vi "SVT Fractional-octave Analysis (N Ch).vi"(0 "scaled signals [EU]":waveform(dbl)[](array[waveform])=[{"t0"=timestamp(0 s since 1904-01-01), "dt"=1.0, "Y"=[]}], 1 "restart averaging (F)":bool, 2 "reset filter (F)":bool, 5 "frequency range [Hz]":T8={"low frequency"=125.0, "high frequency"=8000.0} {"high frequency" min=0.001 format="%.2f"; "low frequency" min=0.001 format="%.2f"}, 7 "bandwidth":T2(ring)=enum."1/12 octave", 9 "dB On (T)":bool=TRUE, 11 "error in (no error)":errorcluster, 12 "averaging type":T9(ring), 13 "exp avg settings":T1={" mode"=enum."Fast", "time constant [ms]"=125.0} {"time constant [ms]" format="%.2f"}, 14 "equal confidence level [dB]":dbl=125.0 format="%.2f") -> (3 "filter settled":bool, 4 "octave spectra":T7(array[cluster]) {"band power" format="%.2f"; "nominal frequencies [Hz]" format="%.2f"}, 6 "unit labels":string[](array[string]), 8 "total band powers":dbl[](array[numeric]) format="%.2f", 10 "octave info":T3[](array[typedef]) {"engineering units" items=["custom..."=0, "V"=1, "A"=21, "C"=30, "pC"=31, "s"=32, "-"=29, "Pa"=2, "N"=20, "g"=3, "m/s^2"=4, "m/s"=5, "m"=6, "mm/s"=12, "mm"=13, "micron/s"=14, "micron"=15, "in/s^2"=7, "in/s"=8, "in"=9, "mil/s"=10, "mil"=11, "rad/s^2"=16, "rad/s"=17, "rad"=18, "deg/s^2"=26, "deg/s"=27, "deg"=28, "RPM"=22, "cycle/s^2"=23, "Hz"=24, "cycle"=25, "strain"=19]; "dB reference" format="%.2e"; "weighting filter" items=["Linear", "A-weighting", "B-weighting", "C-weighting", "ITU-R 468-4", "Dolby", "CCITT", "C-message", "Wb", "Wc", "Wd", "We", "Wf", "Wh", "Wj", "Wk", "Wm", "AES17 20 kHz lowpass", "AES17 40 kHz lowpass", "AES17 20 kHz highpass", "AES17 40 kHz highpass"]}, 15 "error out":errorcluster)   [LabVIEW 2017, in "SoundVib_Octave_2014 standard.lvlib"]
doc: "Performs a fractional-octave analysis on <B>scaled signal [EU]</B> in accordance with the IEC 61260:2014 and ANSI S1.11-2014 standards. Wire data to the <B>scaled signal [EU]</B> input to determine the polymorphic instance to use or manually select the instance."
uses:
  <vilib>/addons/Sound and Vibration/svt_Octave/SoundVib_Octave_2014 standard.lvlib
  <vilib>/addons/_NISVFA/_Shared subVIs/Controls/svc_Octave Info.ctl
  <vilib>/addons/_NISVFA/_Shared subVIs/Controls/svc_Octave Standard.ctl
  <vilib>/addons/_NISVFA/_Shared subVIs/Controls/svc_Weighting Filter Text Ring.ctl
  <vilib>/addons/_NISVFA/_Shared subVIs/Controls/svc_Engineering Units Text Ring.ctl
panel:
  out "# samples to settle":u64
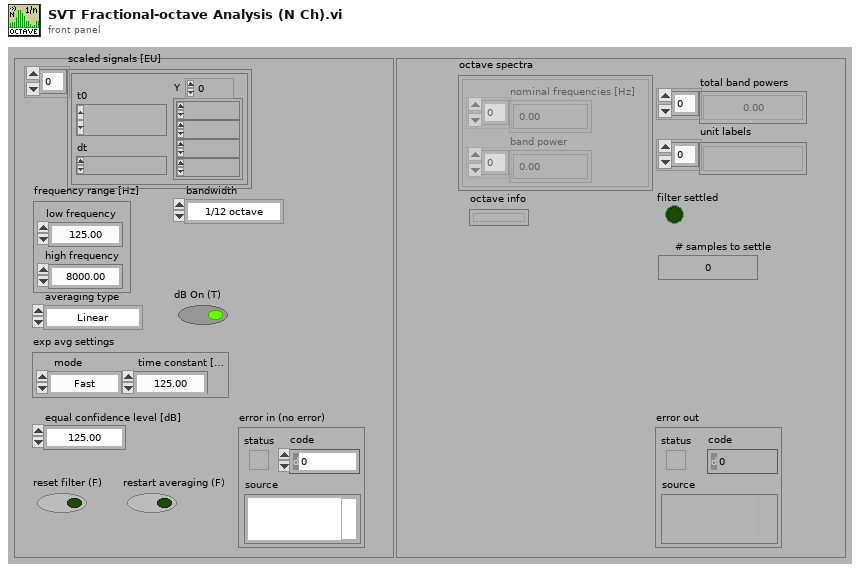
[diagram p1: front panel]
types:
  T1 = cluster{" mode":enum16{"Slow", "Fast", "Impulse", "Custom"}, "time constant [ms]":dbl}
  T2 = enum16{"1 octave", "1/3 octave", "1/6 octave", "1/12 octave", "1/24 octave"}
  T3 = typedef "svc_Octave Info.ctl" = cluster{"standard":T4, "bandwidth":enum16{"1 octave", "1/3 octave", "1/6 octave", "1/12 octave", "1/24 octave"}, "low band":i32, "high band":i32, "weighting filter":T5, "dB reference":dbl, "dB On":bool, "unit label":string, "channel name":string, "description":string, "engineering units":T6, "custom label":string, "spectrum type":enum16{"power", "magnitude"}, "spectral density":bool, "filters settled":bool}
  T4 = typedef "svc_Octave Standard.ctl" = enum16{"ANSI S1.11", "IEC 61260"}
  T5 = typedef "svc_Weighting Filter Text Ring.ctl" = u16
  T6 = typedef "svc_Engineering Units Text Ring.ctl" = u16
  T7 = cluster{"nominal frequencies [Hz]":dbl[], "band power":dbl[]}[]
  T8 = cluster{"low frequency":dbl, "high frequency":dbl}
  T9 = enum16{"Linear", "Exponential", "Equal confidence", "Peak"}
  T10 = cluster{"standard":T4, "bandwidth":enum16{"1 octave", "1/3 octave", "1/6 octave", "1/12 octave", "1/24 octave"}}
  T11 = cluster{"dup nominal frequencies [Hz":dbl[], "band power [EU^2 rms]":dbl[]}[]
  T12 = cluster{"nominal frequencies [Hz]":dbl[], "band power [dB EU]":dbl[]}[]
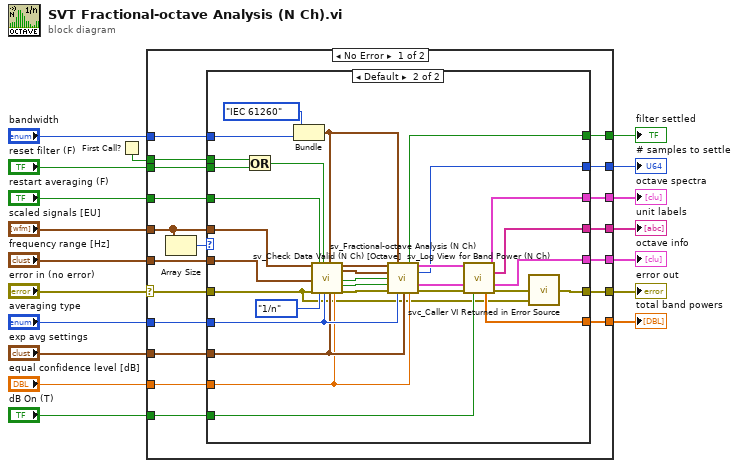
[diagram p0: block diagram]
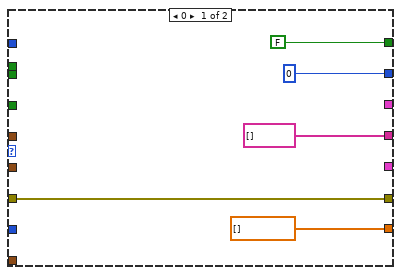
[diagram p2: hidden frame]
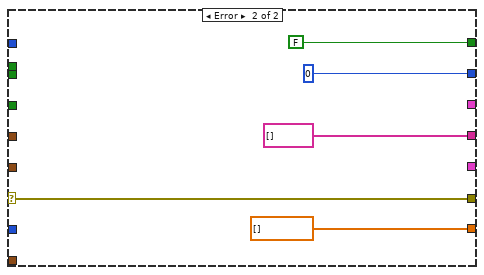
[diagram p3: hidden frame]
diagram:
  n1 = First Call?() -> (First Call?: T/F=w2:bool)
  n2 = case shown="No Error" "error in (no error)" {
    selector: "error in (no error)" -> [w27 w78]
    tunnel: "restart averaging (F)" -> [w37 _]
    tunnel: [w25 FALSE ("settled?")] -> w17
    tunnel: "dB On (T)" -> [w36 _]
    tunnel: "averaging type" -> [w35 _]
    tunnel: [w34 dbl[] [] ("total band power(s) [dB EU]")] -> w14
    tunnel: "equal confidence level [dB]" -> [w26 _]
    tunnel: "bandwidth" -> [w33 _]
    tunnel: "frequency range [Hz]" -> [w32 _]
    tunnel: "exp avg settings" -> [w31 _]
    tunnel: "scaled signals [EU]" -> [w20 _]
    tunnel: [w22 w78] -> w8
    tunnel: [w30 _] -> w7
    tunnel: [w29 _] -> w6
    tunnel: [w28 string[] [] ("unit labels")] -> w5
    tunnel: "reset filter (F)" -> [w24 _]
    tunnel: w2 -> [w23 _]
    tunnel: [w21 u64 0 ("# samples to settle")] -> w1
    frame No Error {
      n3 = Array Size(array=w20) -> (size(s)=w19:i32)
      n4 = case shown="Default" w19 {
        tunnel: w37 -> [_ w73]
        tunnel: w36 -> [_ w68]
        tunnel: w35 -> [_ w66]
        tunnel: [dbl[] [] ("total band power(s) [dB EU]") w65] -> w34
        tunnel: w33 -> [_ w62]
        tunnel: w32 -> [_ w60]
        tunnel: w31 -> [_ w59]
        tunnel: w20 -> [_ w58]
        tunnel: [_ w57] -> w30
        tunnel: [_ w56] -> w29
        tunnel: [string[] [] ("unit labels") w55] -> w28
        tunnel: w27 -> [w41 w43]
        tunnel: w26 -> [_ w51]
        tunnel: [FALSE ("settled?") w49] -> w25
        tunnel: w24 -> [_ w48]
        tunnel: w23 -> [_ w47]
        tunnel: [w41 w45] -> w22
        tunnel: [u64 0 ("# samples to settle") w44] -> w21
        frame 0 {
        }
        frame Default {
          n5 = Or(x=w47, y=w48) -> (x .or. y?=w52:bool)
          n6 = Bundle("standard"=svc_Octave_Standard."IEC 61260", "bandwidth"=w62) -> (w61:T10)  [unwired: 1 in]
          n7 = call <vilib>:"sv_Check Data Valid (N Ch) [Octave].vi"("Scaled signal(s)"=w58, "frequency range [Hz]"=w60, "error in (no error)"=w43, "restart averaging (F)"=w73, "bandwidth"=enum16{"1/1", "1/3", "1/n"}."1/n", "reset filter (F)"=w52, "averaging type"=w66, "1/n Octave settings"=w61, "exp avg settings"=w59, "equal confidence level [dB]"=w51) -> ("dup Scaled signal(s)"=w69:waveform(dbl)[], "band number"=w64:cluster{"low band":i32, "high band":i32}, "Restart averaging"=w71:bool, "Reset Filter"=w50:bool, "error out"=w72:errorcluster)  [unwired: 5 in]
          n8 = call <vilib>:"sv_Fractional-octave Analysis (N Ch).vi"("Scaled signal(s)"=w69, "1/n octave settings"=w61, "band number"=w64, "restart averaging (F)"=w71, "reset filter (F)"=w50, "error in (no error)"=w72, "averaging type"=w66, "exp avg settings"=w59, "equal confidence level [dB]"=w51) -> ("settled?"=w49:bool, "Octave measurements"=w67:T11, "# samples to settle"=w44:u64, "octave info"=w54:T3[], "error out"=w70:errorcluster)  [unwired: 2 in]
          n9 = call <vilib>:"sv_Log View for Band Power (N Ch).vi"("Octave measurements"=w67, "octave info"=w54, "error in (no error)"=w70, "dB On (T)"=w68) -> ("octave spectra"=w56:T12, "unit labels"=w55:string[], "octave info"=w57:T3[], "total band power(s) [dB EU]"=w65:dbl[], "error out"=w46:errorcluster)  [unwired: 7 in]
          n10 = call <vilib>:"svc_Caller VI Returned in Error Source.vi"("warning input to caller"=w43, "error in (no error)"=w46) -> ("error out"=w45:errorcluster)  [unwired: 3 in]
        }
      }
    }
    frame Error {
    }
  }
  "filter settled" <- w17
  "unit labels" <- w5
  "total band powers" <- w14
  "error out" <- w8
  "octave spectra" <- w6
  "octave info" <- w7
  "# samples to settle" <- w1
